vi "Predict.vi"(8 "error in (no error)":errorcluster, 9 "U":T2, 10 "SLAM In":T1) -> (0 "error out":errorcluster, 2 "SLAM Out":T1)   [LabVIEW 2009]
uses:
  Controls/SLAM.ctl
  <vilib>/Analysis/Matrix/Datatypes/RealMatrix.ctl
  <vilib>/Analysis/Matrix/Numeric/Add/Add - RM,RM.vi
  <vilib>/Analysis/baseanly.llb/Real A x B.vi
  <vilib>/Analysis/7linalg.llb/Real Transpose Matrix.vi
  <vilib>/Analysis/NI_AALBase.lvlib
  <vilib>/Analysis/Matrix/NI_Matrix.lvlib
  <vilib>/Analysis/NI_AALPro.lvlib
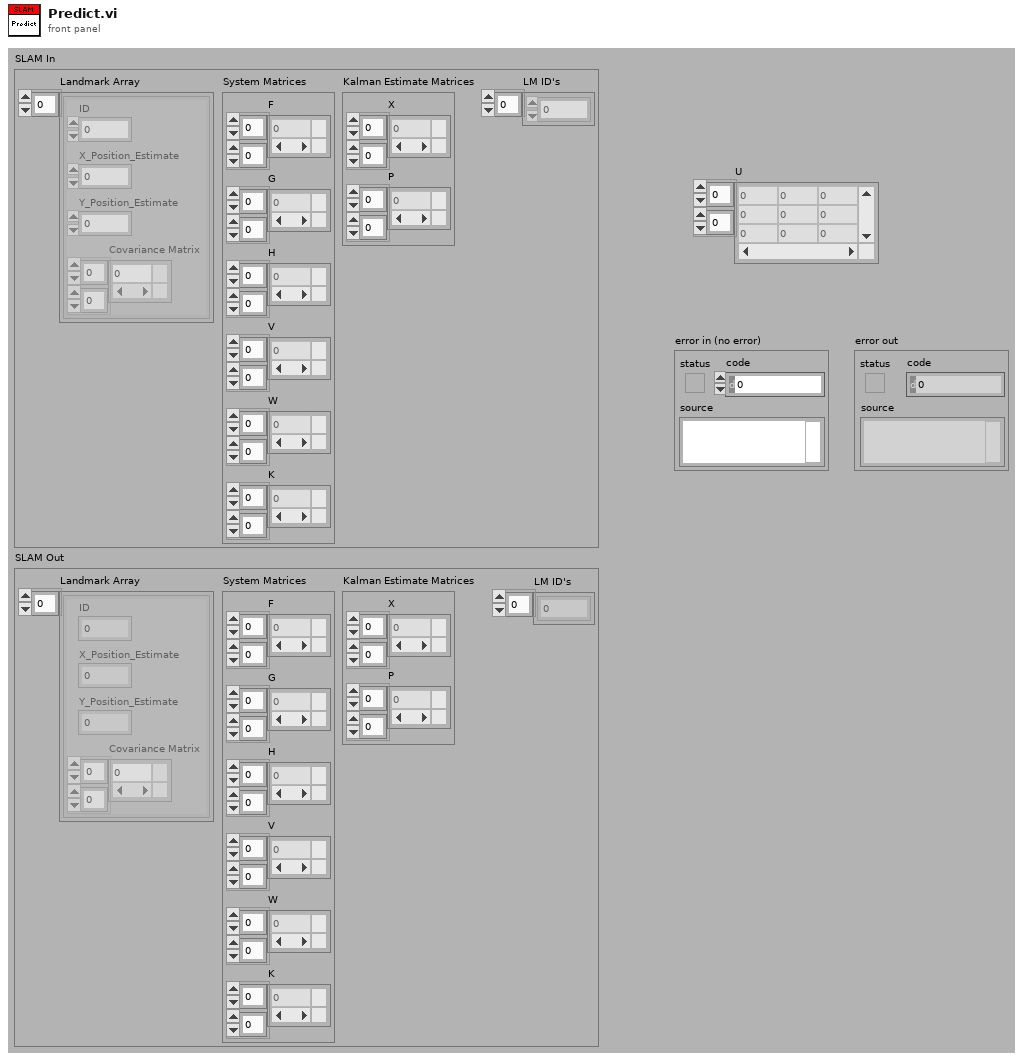
[diagram p1: front panel]
types:
  T1 = typedef "SLAM.ctl" = cluster{"Landmark Array":cluster{"ID":dbl, "X_Position_Estimate":dbl, "Y_Position_Estimate":dbl, "Covariance Matrix":T2}[], "System Matrices":cluster{"F":T2, "G":T2, "H":T2, "V":T2, "W":T2, "K":T2}, "Kalman Estimate Matrices":cluster{"X":T2, "P":T2}, "LM ID's":dbl[]}
  T2 = typedef "NI_Matrix.lvlib/RealMatrix.ctl" = dbl[][]
  T3 = cluster{"F":T2, "G":T2, "H":T2, "V":T2, "W":T2, "K":T2}
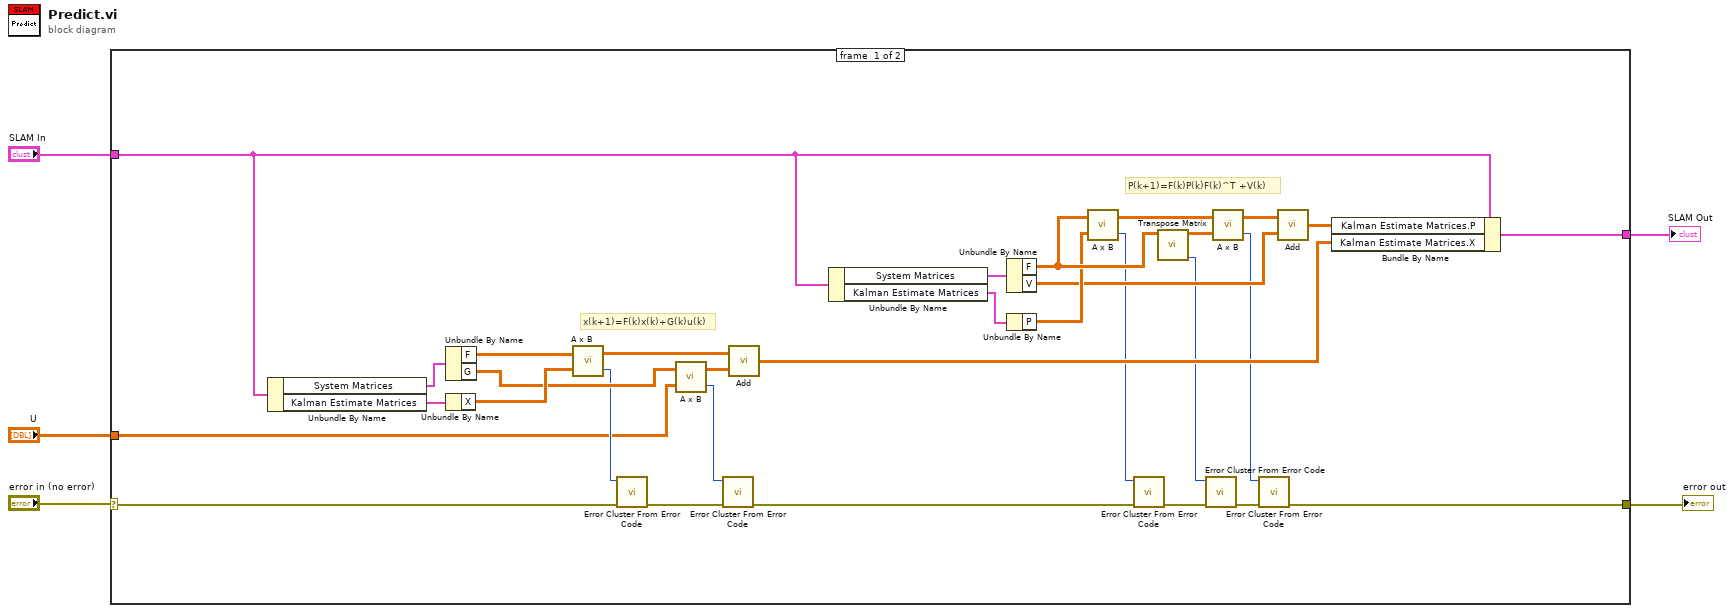
[diagram p0: block diagram]
diagram:
  n1 = case shown="No Error" "error in (no error)" {
    selector: "error in (no error)" -> [w17 w38]
    tunnel: [w9 w38] -> w4
    tunnel: "SLAM In" -> [w8 w37]
    tunnel: "U" -> [w7 _]
    tunnel: [w6 w37] -> w1
    frame #0 {
      # "P(k+1)=F(k)P(k)F(k)^T +V(k)"
      # "x(k+1)=F(k)x(k)+G(k)u(k)"
      n2 = Unbundle By Name(w8) -> ("System Matrices"=w35:T3, "Kalman Estimate Matrices"=w36:cluster{"X":T2, "P":T2})
      n3 = Unbundle By Name(w35) -> ("F"=w32:T2, "G"=w30:T2)
      n4 = Unbundle By Name(w36) -> ("X"=w31:T2)
      n5 = call-poly <vilib>:"A x B.vi"("B"=w31, "A"=w32) -> ("error"=w19:i32, "A x B"=w34:T2)
      n6 = call <vilib>:"Error Cluster From Error Code.vi"("error in (no error)"=w17, "error code (0)"=w19) -> ("error out"=w16:errorcluster)  [unwired: 7 in]
      n7 = call-poly <vilib>:"A x B.vi"("B"=w7, "A"=w30) -> ("error"=w18:i32, "A x B"=w33:T2)
      n8 = call <vilib>:"Error Cluster From Error Code.vi"("error in (no error)"=w16, "error code (0)"=w18) -> ("error out"=w11:errorcluster)  [unwired: 7 in]
      n9 = call-poly <vilib>:"Add.vi"("Real Matrix B"=w33, "Real Matrix A"=w34) -> ("A + B"=w20:T2)
      n10 = Unbundle By Name(w8) -> ("System Matrices"=w22:T3, "Kalman Estimate Matrices"=w26:cluster{"X":T2, "P":T2})
      n11 = Unbundle By Name(w22) -> ("F"=w25:T2, "V"=w23:T2)
      n12 = Unbundle By Name(w26) -> ("P"=w24:T2)
      n13 = call-poly <vilib>:"A x B.vi"("B"=w24, "A"=w25) -> ("error"=w14:i32, "A x B"=w28:T2)
      n14 = call <vilib>:"Error Cluster From Error Code.vi"("error in (no error)"=w11, "error code (0)"=w14) -> ("error out"=w15:errorcluster)  [unwired: 7 in]
      n15 = call-poly <vilib>:"Transpose Matrix.vi"("Input Matrix"=w25) -> ("error"=w13:i32, "Matrix Transpose"=w27:T2)  [unwired: 9 in]
      n16 = call <vilib>:"Error Cluster From Error Code.vi"("error in (no error)"=w15, "error code (0)"=w13) -> ("error out"=w10:errorcluster)  [unwired: 7 in]
      n17 = call-poly <vilib>:"A x B.vi"("B"=w27, "A"=w28) -> ("error"=w12:i32, "A x B"=w29:T2)
      n18 = call <vilib>:"Error Cluster From Error Code.vi"("error in (no error)"=w10, "error code (0)"=w12) -> ("error out"=w9:errorcluster)  [unwired: 7 in]
      n19 = call-poly <vilib>:"Add.vi"("Real Matrix B"=w23, "Real Matrix A"=w29) -> ("A + B"=w21:T2)
      n20 = Bundle By Name(cluster=w8, "Kalman Estimate Matrices.P"=w21, "Kalman Estimate Matrices.X"=w20) -> (w6:T1)
    }
    frame #1 {
    }
  }
  "error out" <- w4
  "SLAM Out" <- w1
